vi "Send Message.vi"(0 "MLA":refnum<class "MLA.lvclass">, 1 "Message":string, 2 "Param 1":string, 3 "Param 2":string, 4 "Params":string[](array[string]), 5 "error in (no error)":errorcluster) -> (14 "MLA":refnum<class "MLA.lvclass">, 19 "error out":errorcluster)   [LabVIEW 2017, in "MLA.lvclass"]
uses:
  MLA.lvclass
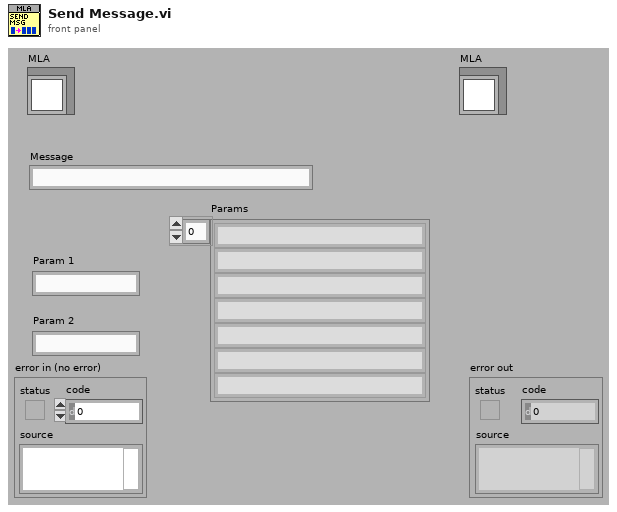
[diagram p1: front panel]
types:
  T1 = typedef "MLA.lvclass/ObjectAttributes.ctl" = cluster{"App Name":string, "App Version":string, "Revision History":string, "Log File Path":path, "Config INI File":path, "Config Path":path, "Log Archive Path":path, "Msg Q's":refnum<queue>[], "VI":refnum<vi>, "ErrLog":refnum<class "ErrorLog.lvclass">}
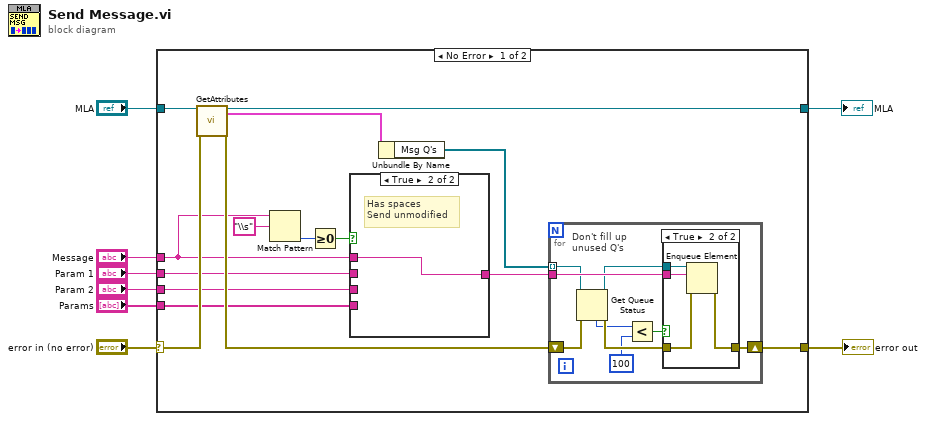
[diagram p0: block diagram]
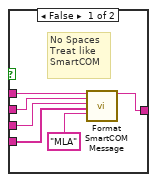
[diagram p2: hidden frame]
diagram:
  n1 = case shown="No Error" "error in (no error)" {
    selector: "error in (no error)" -> [w23 w46]
    tunnel: [w17 w46] -> w7
    tunnel: [w20 w45] -> w5
    tunnel: "MLA" -> [w21 w45]
    tunnel: "Message" -> [w12 _]
    tunnel: "Param 1" -> [w15 _]
    tunnel: "Param 2" -> [w14 _]
    tunnel: "Params" -> [w13 _]
    frame No Error {
      n2 = call "GetAttributes.vi"("MLA"=w21, "error in (no error)"=w23) -> ("MLA"=w20:refnum<class "MLA.lvclass">, "Data"=w22:T1, "error out"=w18:errorcluster)  [unwired: 14 in, 1 out]
      n3 = Match Pattern(string=w12, regular expression="\\s") -> (offset past match=w10:i32)  [unwired: 1 in, 3 out]
      n4 = Greater Or Equal To 0?(x=w10) -> (x >= 0?=w9:bool)
      n5 = case shown="True" w9 {
        tunnel: [w29 w30] -> w16
        tunnel: w15 -> [w28 _]
        tunnel: w14 -> [w27 _]
        tunnel: w13 -> [w26 _]
        tunnel: w12 -> [w24 w30]
        frame False {
          # "No Spaces\nTreat like\nSmartCOM"
          n6 = call "Format SmartCOM Message.vi"("Message"=w24, "Param 1"=w28, "Param 2"=w27, "Params"=w26, "Name"="MLA") -> ("Message to Send"=w29:string)  [unwired: 14 in]
        }
        frame True {
          # "Has spaces\nSend unmodified"
        }
      }
      n7 = Unbundle By Name(w22) -> ("Msg Q's"=w19:refnum<queue>[])
      n8 = for {
        tunnel: w19 -> [w37] mode=indexing
        tunnel: w16 -> [w39]
        shift-right: [w38] -> w17
        shift-left: w18 -> [w35]
        # "Don't fill up unused Q's"
        n9 = Get Queue Status(queue=w37, error in (no error)=w35) -> (queue out=w36:refnum<queue>, error out=w34:errorcluster, # elements in queue=w33:i32)  [unwired: 1 in, 5 out]
        n10 = Less?(x=w33, y=100) -> (x < y?=w31:bool)
        n11 = case shown="True" w31 {
          tunnel: w39 -> [_ w44]
          tunnel: w34 -> [w40 w43]
          tunnel: [w40 w42] -> w38
          tunnel: w36 -> [_ w41]
          frame False {
          }
          frame True {
            n12 = Enqueue Element(queue=w41, element=w44, error in (no error)=w43) -> (error out=w42:errorcluster)  [unwired: 1 in, 2 out]
          }
        }
      }
    }
    frame Error {
    }
  }
  "error out" <- w7
  "MLA" <- w5
